vi "Load.vi"(8 "Error in":errorcluster, 11 "Vi Path":path=path "C:/Users/namratha.balakrishna/Documents/LabVIEW Data/MDI/source code/Labview MDI/Example/Waveform.vi") -> (0 "Error Out":errorcluster, 3 "MDI.lvlib:Document.lvclass":refnum<class "Document.lvclass">)   [LabVIEW 2016, in "Document.lvclass"]
uses:
  Document.lvclass
  Document.lvclass/Document.ctl
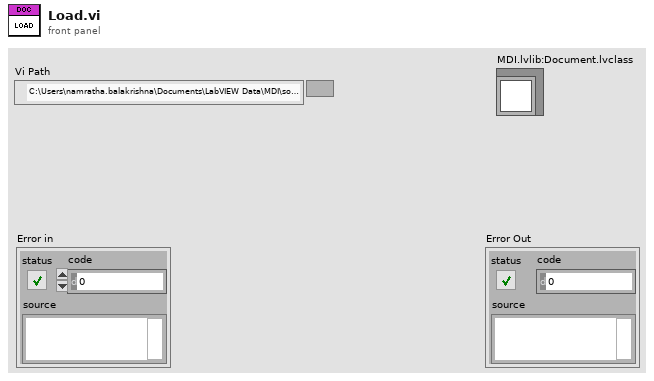
[diagram p1: front panel]
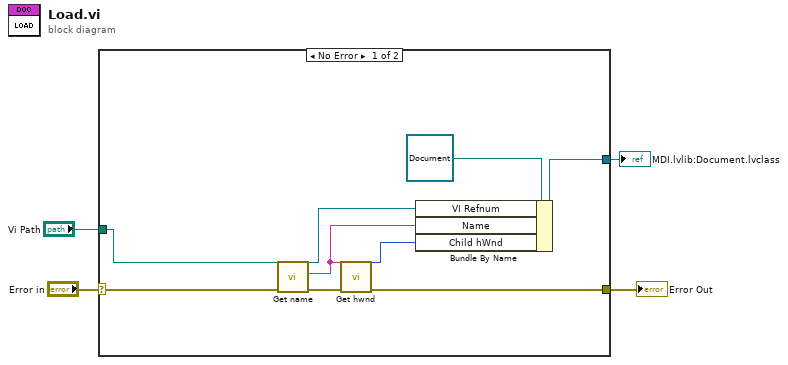
[diagram p0: block diagram]
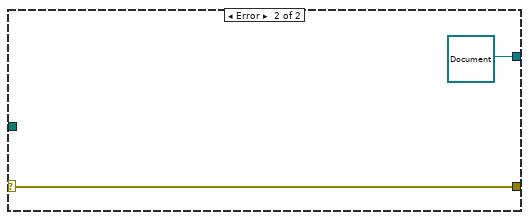
[diagram p2: hidden frame]
diagram:
  n1 = case shown="No Error" "Error in" {
    selector: "Error in" -> [w11 w15]
    tunnel: [w13 w15] -> w3
    tunnel: "Vi Path" -> [w12 _]
    tunnel: [w10 refnum<class "Document.lvclass"> refnum ("MDI.lvlib:Document.lvclass")] -> w1
    frame No Error {
      n2 = call "Get name.vi"("Error in"=w11, "Vi Path"=w12) -> ("Error Out"=w9:errorcluster, "Name"=w5:string, "vi reference"=w8:refnum<vi>)  [unwired: 7 in]
      n3 = call "Get hwnd.vi"("Error in"=w9, "Name"=w5) -> ("Error Out"=w13:errorcluster, "hwnd"=w7:u32)  [unwired: 8 in]
      n4 = Bundle By Name(cluster=refnum<class "Document.lvclass"> refnum ("MDI.lvlib:Document.lvclass"), "VI Refnum"=w8, "Name"=w5, "Child hWnd"=w7) -> (w10:refnum<class "Document.lvclass">)
    }
    frame Error {
    }
  }
  "Error Out" <- w3
  "MDI.lvlib:Document.lvclass" <- w1
